vi "Start Server.vi"(5 "Server Key File (.key)":path, 7 "Server Certificate File (.crt)":path, 8 "error in":errorcluster, 10 "gRPCid server in":T1, 11 "Server Address":string) -> (0 "error out":errorcluster, 2 "Listening Port":i32, 3 "gRPCid server out":T1)   [LabVIEW 2019, in "grpc-lvsupport.lvlib"]
uses:
  grpc-lvsupport.lvlib
  grpcId.ctl
  <vilib>/Utility/file.llb/Application Directory.vi
  <vilib>/Utility/error.llb/Error Cluster From Error Code.vi
  <resource>/labview_grpc_server.dll
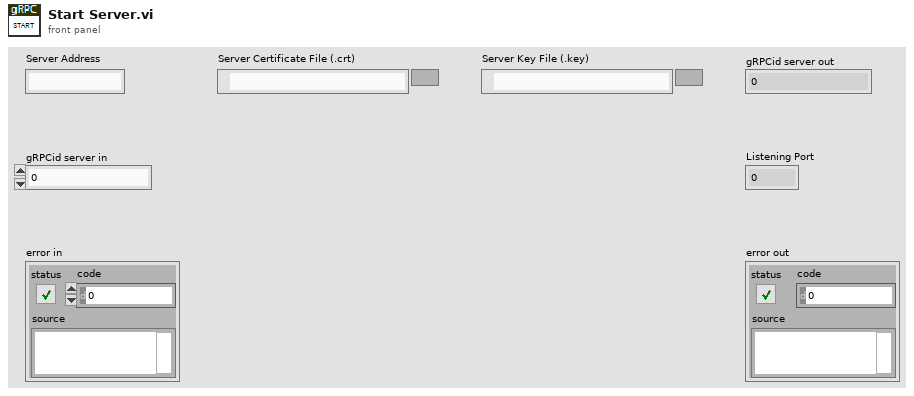
[diagram p1: front panel]
types:
  T1 = typedef "grpc-lvsupport.lvlib/grpcId.ctl" = u64
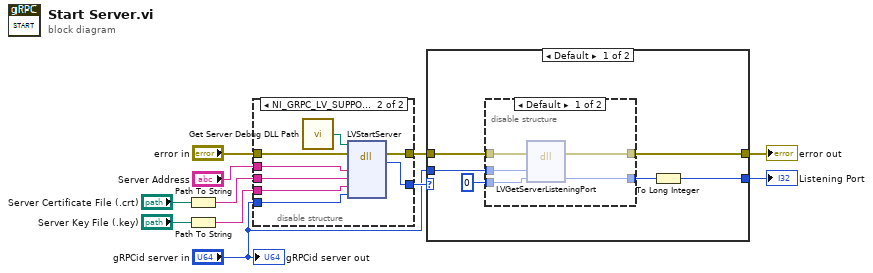
[diagram p0: block diagram]
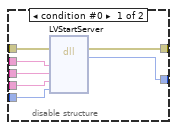
[diagram p2: hidden frame]
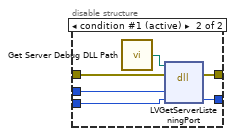
[diagram p3: hidden frame]
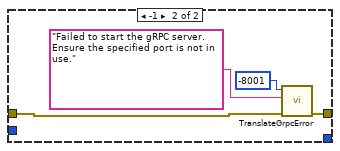
[diagram p4: hidden frame]
diagram:
  n1 = Path To String(path="Server Certificate File (.crt)") -> (string=w8:string)
  n2 = Path To String(path="Server Key File (.key)") -> (string=w7:string)
  n3 = disable-structure shown="NI_GRPC_LV_SUPPORT_DEBUG==True&&RUN_TIME_ENGINE==False" {
    disable-tunnel: "error in" -> [w18 w26]
    disable-tunnel: [w17 w25] -> w10
    disable-tunnel: "Server Address" -> [w16 w24]
    disable-tunnel: w8 -> [w15 w23]
    disable-tunnel: w7 -> [w14 w22]
    disable-tunnel: [w13 w21] -> w4
    disable-tunnel: "gRPCid server in" -> [w12 w19]
    frame condition #0 {
      n4 = dll-call lib="C:/Program Files (x86)/National Instruments/LabVIEW 2024/resource/labview_grpc_server.*" fn="LVStartServer"(error in=w18, "serveraddress"=w16, "serverCertificateFile"=w15, "serverKeyFile"=w14, "serverid"=w12) -> (error out=w17:errorcluster, "return type"=w13:i32)  [unwired: 6 in, 1 out]
    }
    frame condition #1 (active) {
      n5 = call "Get Server Debug DLL Path.vi"() -> ("DLL Path"=w20:path)
      n6 = dll-call lib="?" fn="LVStartServer"(path in=w20, error in=w26, "serveraddress"=w24, "serverCertificateFile"=w23, "serverKeyFile"=w22, "serverid"=w19) -> (error out=w25:errorcluster, "return type"=w21:i32)  [unwired: 5 in, 1 out]
    }
  }
  n7 = case shown="Default" w4 {
    tunnel: [w32 w44] -> w2
    tunnel: w10 -> [w31 w47]
    tunnel: "gRPCid server in" -> [w30 _]
    tunnel: [w27 _] -> w1
    frame Default {
      n8 = disable-structure shown="Default" {
        disable-tunnel: [w37 w43] -> w32
        disable-tunnel: w31 -> [w36 w42]
        disable-tunnel: w30 -> [w35 w41]
        disable-tunnel: [w34 w40] -> w29
        disable-tunnel: u64 0 ("listeningPort") -> [w33 w39]
        frame condition #0 {
          n9 = dll-call lib="C:/Program Files (x86)/National Instruments/LabVIEW 2024/resource/labview_grpc_server.*" fn="LVGetServerListeningPort"(error in=w36, "serverId"=w35, "listeningPort"=w33) -> (error out=w37:errorcluster, "listeningPort"=w34:i64)  [unwired: 4 in, 1 out]
        }
        frame condition #1 (active) {
          n10 = call "Get Server Debug DLL Path.vi"() -> ("DLL Path"=w38:path)
          n11 = dll-call lib="?" fn="LVGetServerListeningPort"(path in=w38, error in=w42, "serverId"=w41, "listeningPort"=w39) -> (error out=w43:errorcluster, "listeningPort"=w40:i64)  [unwired: 3 in, 1 out]
        }
      }
      n12 = To Long Integer(number=w29) -> (32bit integer=w27:i32)
    }
    frame -1 {
      n13 = call "TranslateGrpcError.vi"("error in"=w47, "Error Message"="Failed to start the gRPC server.  Ensure the specified port is not in use.", "Error Code"=-8001) -> ("error out"=w44:errorcluster)  [unwired: 8 in]
    }
  }
  "error out" <- w2
  "Listening Port" <- w1
  "gRPCid server out" <- "gRPCid server in"
